vi "Queue Name.vi"(11 "Remote VI Queue in":refnum<queue>) -> (2 "Queue Name":string, 3 "Remote VI Queue out":refnum<queue>)   [LabVIEW 2020, in "Dynamic Reentrant.lvlib"]
uses:
  <userlib>/DynamicReentrant/Dynamic Reentrant.lvlib
  <userlib>/DynamicReentrant/src/Type Defs/Message.ctl
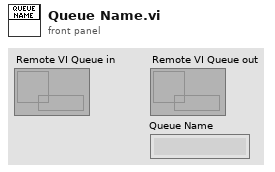
[diagram p1: front panel]
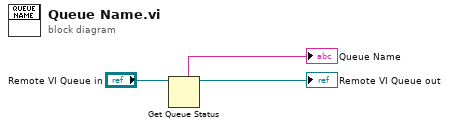
[diagram p0: block diagram]
diagram:
  n1 = Get Queue Status(queue="Remote VI Queue in") -> (queue out=→"Remote VI Queue out":refnum<queue>, queue name=→"Queue Name":string)  [unwired: 2 in, 6 out]
